vi "Untitled 9.vi"() -> ()   [LabVIEW 2016]
uses:
  <userlib>/LevyLab/Levylab Instruments/Instrument Types/Cryostat/Instrument.Cryostat.lvclass
panel:
  out "class name":string
  out "specific class reference":refnum<class "Instrument.Cryostat.lvclass">
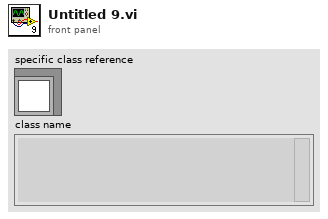
[diagram p1: front panel]
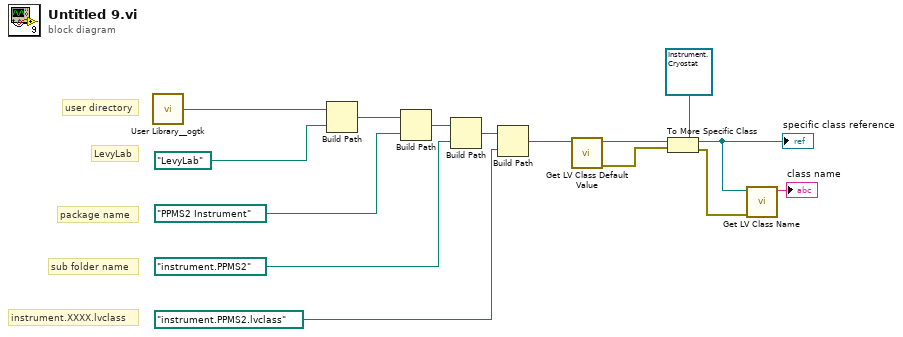
[diagram p0: block diagram]
diagram:
  # "LevyLab"
  # "user directory"
  # "instrument.XXXX.lvclass"
  # "sub folder name"
  # "package name"
  n1 = call <userlib>:"User Library__ogtk.vi"() -> ("User Library (+ Relative)"=w13:path)  [unwired: 1 in]
  n2 = Build Path(base path=w13, name or relative path=path "LevyLab" ("class path")) -> (appended path=w12:path)
  n3 = Build Path(base path=w12, name or relative path=path "PPMS2 Instrument" ("class path")) -> (appended path=w11:path)
  n4 = Build Path(base path=w11, name or relative path=path "instrument.PPMS2" ("class path")) -> (appended path=w10:path)
  n5 = Build Path(base path=w10, name or relative path=path "instrument.PPMS2.lvclass" ("class path")) -> (appended path=w9:path)
  n6 = call <vilib>:"Get LV Class Default Value.vi"("class path"=w9) -> ("error out"=w14:errorcluster, "object"=w15:refnum<class>)  [unwired: 9 in]
  n7 = To More Specific Class(target class=refnum<class "Instrument.Cryostat.lvclass"> refnum ("Instrument.Cryostat in"), reference=w15, error in=w14) -> (specific class reference=w3:refnum<class "Instrument.Cryostat.lvclass">, error out=w1:errorcluster)
  "specific class reference" <- w3
  n8 = call <vilib>:"Get LV Class Name.vi"("error in (no error)"=w1, "object"=w3) -> ("class name"=→"class name":string)  [unwired: 8 in, 1 out]
